vi "LTE Example.vi"() -> ()   [LabVIEW 2016]
uses:
  Source/SA/RFmxLTE/Typedefs/LTE Common Configuration.ctl
  Source/SA/RFmxLTE/Typedefs/LTE Signal Configuration.ctl
  Source/SA/RFmxLTE/Typedefs/LTE Component Carrier Configuration.ctl
  Source/SA/RFmxLTE/Typedefs/LTE ModAcc Configuration.ctl
  Source/SA/RFmxLTE/Typedefs/LTE ACP Configuration.ctl
  Source/SA/RFmxLTE/Typedefs/LTE ModAcc Results.ctl
  Source/SA/RFmxLTE/Typedefs/LTE ModAcc Component Carrier Results.ctl
  Source/SA/RFmxLTE/Typedefs/LTE ACP Results.ctl
  Source/SA/RFmxLTE/Typedefs/LTE ACP Offset Results.ctl
  Source/SA/RFmxLTE/Typedefs/LTE ACP Component Carrier Results.ctl
  Source/SA/RFmxLTE/RFmxLTE.lvlib
panel:
  out "error out":errorcluster
  out "ACP Results":T1
  out "ModAcc Results":T4
  in  "Tab Control":enum32{"Common", "Signal", "ACP", "ModAcc"}(tab)
  in  "Common Configuration":T6={"Center Frequency (Hz)"=1000000000.0, "Reference Level (dBm)"=0.0, "External Attenuation (dB)"=0.0, "Frequency Reference Source"="OnboardClock", "Enable Trigger?"=TRUE, "Digital Edge Source"="PXI_Trig0", "Digital Edge"=0, "Trigger Delay (s)"=0.0} {"External Attenuation (dB)" format="%.2f"; "Reference Level (dBm)" format="%.2f"; "Center Frequency (Hz)" format="%.6p"; "Trigger Delay (s)" format="%.3p"; "Digital Edge" items=["Rising Edge", "Falling Edge"]}
  in  "Resource Name":refnum<k15>="VST"
  in  "LTE Signal Configuration":T7={"Link Direction"=1, "Duplex Scheme"=0, "Uplink Downlink Configuration"=0, "Band"=1, "PUSCH Auto Resource Block Detection Enabled"=1, "Auto DMRS Detection Enabled"=0, "DL Auto Cell ID Detection Enabled"=0, "CC Configuration"=[{"Bandwidth (Hz)"=10000000.0, "Cell ID"=0, "PUSCH Modulation Type"=0, "PUSCH Resource Block Offset"=0, "PUSCH Number of Resource Blocks"=-1, "DL Test Model"=0}]} {"DL Auto Cell ID Detection Enabled" items=["False", "True"]; "Link Direction" items=["FDD", "TDD", "LAA"]; "Auto DMRS Detection Enabled" items=["False", "True"]; "PUSCH Auto Resource Block Detection Enabled" items=["False", "True"]; "CC Configuration"."DL Test Model" items=["TM1.1", "TM1.2", "TM2", "TM 2a", "TM 3.1", "TM 3.2", "TM 3.3", "TM 3.1a"]; "CC Configuration"."PUSCH Modulation Type" items=["QPSK", "16 QAM", "64 QAM", "256 QAM", "1024 QAM"]; "CC Configuration"."Bandwidth (Hz)" items=["200.0 k"=200000.0, "1.4 M"=1400000.0, "3.0 M"=3000000.0, "5.0 M"=5000000.0, "10.0 M"=10000000.0, "15.0 M"=15000000.0, "20.0 M"=20000000.0]; "Uplink Downlink Configuration" items=["0", "1", "2", "3", "4", "5", "6"]; "Duplex Scheme" items=["0", "1", "2", "3", "4", "5", "6"]}
  in  "ACP Configuration":T9={"Measurement Enabled"=TRUE, "Number of GSM Offsets"=0, "Number of UTRA Offsets"=2, "Number of EUTRA Offsets"=1, "Sweep Time Auto"=1, "Sweep Time Interval (s)"=0.001, "Averaging Enabled"=0, "Averaging Count"=10, "Averaging Type"=0, "RBW Auto"=1, "RBW (Hz)"=30000.0, "RBW Filter Type"=0} {"RBW Filter Type" items=["FFT Based", "Gaussian", "Flat"]; "RBW Auto" items=["False", "True"]; "Averaging Type" items=["RMS", "Log", "Scalar", "Max", "Min"]; "Averaging Enabled" items=["False", "True"]; "Sweep Time Auto" items=["False", "True"]}
  in  "ModAcc Configuration":T10={"Measurement Enabled"=TRUE, "Synchronization Mode"=1, "Measurement Offset (slots)"=0, "Measurement Length (slots)"=1, "EVM Unit"=0, "Averaging Enabled"=0, "Averaging Count"=10} {"Averaging Enabled" items=["False", "True"]; "EVM Unit" items=["Percentage", "dB"]; "Synchronization Mode" items=["Frame", "Slot", "Marker"]}
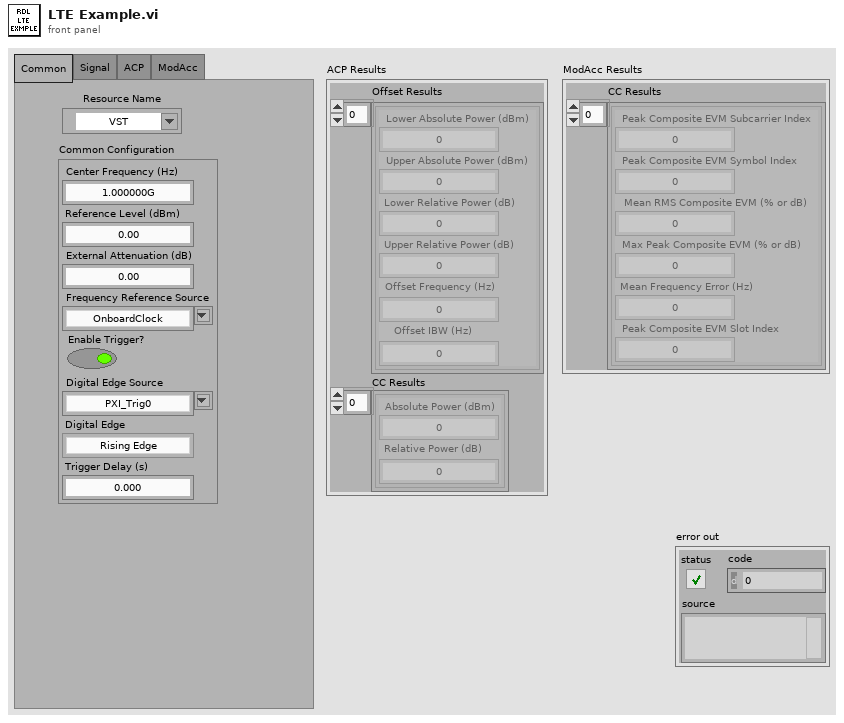
[diagram p1: front panel]
types:
  T1 = typedef "RFmxLTE.lvlib/LTE ACP Results.ctl" = cluster{"Offset Results":T2[], "CC Results":T3[]}
  T2 = typedef "RFmxLTE.lvlib/LTE ACP Offset Results.ctl" = cluster{"Lower Absolute Power (dBm)":dbl, "Upper Absolute Power (dBm)":dbl, "Lower Relative Power (dB)":dbl, "Upper Relative Power (dB)":dbl, "Offset Frequency (Hz)":dbl, "Offset IBW (Hz)":dbl}
  T3 = typedef "RFmxLTE.lvlib/LTE ACP Component Carrier Results.ctl" = cluster{"Absolute Power (dBm)":dbl, "Relative Power (dB)":dbl}
  T4 = typedef "RFmxLTE.lvlib/LTE ModAcc Results.ctl" = cluster{"CC Results":T5[]}
  T5 = typedef "RFmxLTE.lvlib/LTE ModAcc Component Carrier Results.ctl" = cluster{"Peak Composite EVM Subcarrier Index":i32, "Peak Composite EVM Symbol Index":i32, "Mean RMS Composite EVM (% or dB)":dbl, "Max Peak Composite EVM (% or dB)":dbl, "Mean Frequency Error (Hz)":dbl, "Peak Composite EVM Slot Index":i32}
  T6 = typedef "RFmxLTE.lvlib/LTE Common Configuration.ctl" = cluster{"Center Frequency (Hz)":dbl, "Reference Level (dBm)":dbl, "External Attenuation (dB)":dbl, "Frequency Reference Source":string, "Enable Trigger?":bool, "Digital Edge Source":string, "Digital Edge":i32, "Trigger Delay (s)":dbl}
  T7 = typedef "RFmxLTE.lvlib/LTE Signal Configuration.ctl" = cluster{"Link Direction":i32, "Duplex Scheme":i32, "Uplink Downlink Configuration":i32, "Band":i32, "PUSCH Auto Resource Block Detection Enabled":i32, "Auto DMRS Detection Enabled":i32, "DL Auto Cell ID Detection Enabled":i32, "CC Configuration":T8[]}
  T8 = typedef "RFmxLTE.lvlib/LTE Component Carrier Configuration.ctl" = cluster{"Bandwidth (Hz)":dbl, "Cell ID":i32, "PUSCH Modulation Type":i32, "PUSCH Resource Block Offset":i32, "PUSCH Number of Resource Blocks":i32, "DL Test Model":i32}
  T9 = typedef "RFmxLTE.lvlib/LTE ACP Configuration.ctl" = cluster{"Measurement Enabled":bool, "Number of GSM Offsets":i32, "Number of UTRA Offsets":i32, "Number of EUTRA Offsets":i32, "Sweep Time Auto":i32, "Sweep Time Interval (s)":dbl, "Averaging Enabled":i32, "Averaging Count":i32, "Averaging Type":i32, "RBW Auto":i32, "RBW (Hz)":dbl, "RBW Filter Type":i32}
  T10 = typedef "RFmxLTE.lvlib/LTE ModAcc Configuration.ctl" = cluster{"Measurement Enabled":bool, "Synchronization Mode":i32, "Measurement Offset (slots)":i32, "Measurement Length (slots)":i32, "EVM Unit":i32, "Averaging Enabled":i32, "Averaging Count":i32}
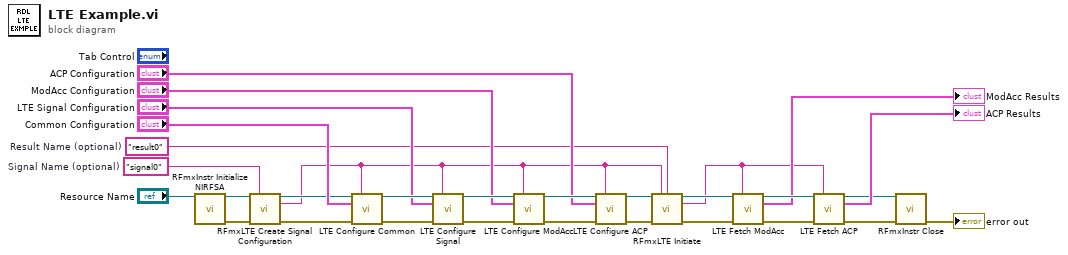
[diagram p0: block diagram]
diagram:
  w2 = "result0"  # Result Name (optional)
  w4 = "signal0"  # Signal Name (optional)
  n1 = call <vilib>:"RFmxInstr Initialize NIRFSA.vi"("Resource Name"="Resource Name") -> ("Instrument Handle Out"=w6:refnum<k21>, "error out"=w28:errorcluster)  [unwired: 12 in, 1 out]
  n2 = call <vilib>:"RFmxLTE Create Signal Configuration.vi"("Instrument Handle In"=w6, "Signal Name"=w4, "error in (no error)"=w28) -> ("Instrument Handle Out"=w5:refnum<k21>, "Selector String Out"=w3:string, "error out"=w7:errorcluster)  [unwired: 10 in]
  n3 = call "LTE Configure Common.vi"("Instrument Handle In"=w5, "Selector String"=w3, "Common Configuration"="Common Configuration", "error in (no error)"=w7) -> ("Instrument Handle Out"=w30:refnum<k21>, "error out"=w29:errorcluster)  [unwired: 10 in]
  n4 = call "LTE Configure Signal.vi"("Instrument Handle In"=w30, "Selector String"=w3, "LTE Signal Configuration"="LTE Signal Configuration", "error in (no error)"=w29) -> ("Instrument Handle Out"=w24:refnum<k21>, "error out"=w23:errorcluster)  [unwired: 10 in]
  n5 = call "LTE Configure ModAcc.vi"("RFmx Handle In"=w24, "Selector String"=w3, "RFmx LTE ModAcc Configuration"="ModAcc Configuration", "error in (no error)"=w23) -> ("RFmx Handle Out"=w22:refnum<k21>, "error out"=w21:errorcluster)  [unwired: 10 in]
  n6 = call "LTE Configure ACP.vi"("RFmx Handle In"=w22, "Selector String"=w3, "RFmx LTE ACP Configuration"="ACP Configuration", "error in (no error)"=w21) -> ("RFmx Handle Out"=w19:refnum<k21>, "error out"=w18:errorcluster)  [unwired: 10 in]
  n7 = call <vilib>:"RFmxLTE Initiate.vi"("Instrument Handle In"=w19, "Selector String"=w3, "Result Name"=w2, "error in (no error)"=w18) -> ("Instrument Handle Out"=w16:refnum<k21>, "Selector String Out"=w8:string, "error out"=w15:errorcluster)  [unwired: 9 in]
  n8 = call "LTE Fetch ModAcc.vi"("RFmx Handle In"=w16, "Selector String"=w8, "error in (no error)"=w15) -> ("RFmx Handle Out"=w14:refnum<k21>, "ModAcc Results"=→"ModAcc Results":T4, "error out"=w1:errorcluster)  [unwired: 10 in]
  n9 = call "LTE Fetch ACP.vi"("RFmx Handle In"=w14, "Selector String"=w8, "error in (no error)"=w1) -> ("RFmx Handle Out"=w11:refnum<k21>, "ACP Results"=→"ACP Results":T1, "error out"=w10:errorcluster)  [unwired: 10 in]
  n10 = call <vilib>:"RFmxInstr Close.vi"("Instrument Handle In"=w11, "error in (no error)"=w10) -> ("error out"=→"error out":errorcluster)  [unwired: 13 in]
